vi "Acquire.vi"(8 "error in (no error)":errorcluster, 11 "Sensor in":refnum<class "Sensor.lvclass">) -> (0 "error out":errorcluster, 3 "Sensor out":refnum<class "Sensor.lvclass">)   [LabVIEW 2012, in "Sensor Definition.lvlib" / "Sensor.lvclass"]
uses:
  Sensor.lvclass
  Double Scalar SensorData.lvclass
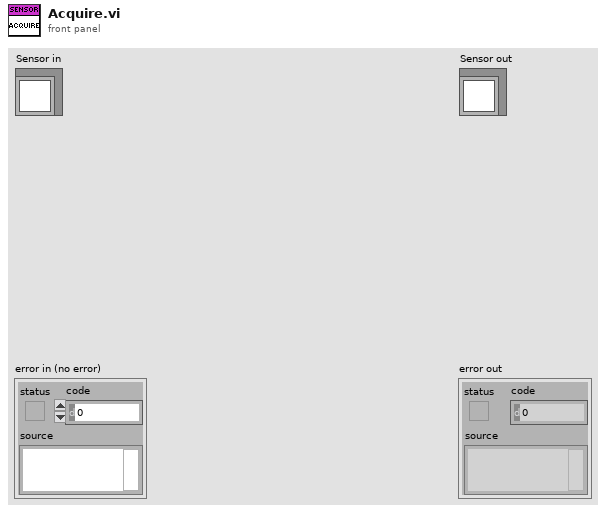
[diagram p1: front panel]
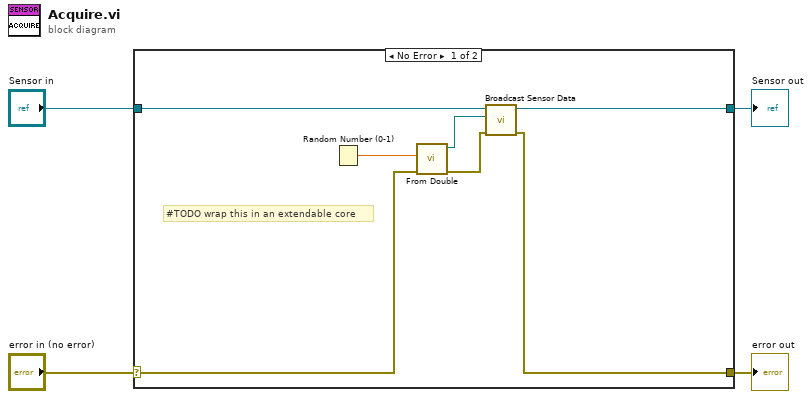
[diagram p0: block diagram]
diagram:
  n1 = case shown="No Error" "error in (no error)" {
    selector: "error in (no error)" -> [w6 w13]
    tunnel: [w9 w13] -> w3
    tunnel: [w10 w12] -> w1
    tunnel: "Sensor in" -> [w11 w12]
    frame No Error {
      # "#TODO wrap this in an extendable core"
      n2 = Random Number (0-1)() -> (number: 0 to 1=w7:dbl)
      n3 = call "From Double.vi"("error in (no error)"=w6, "Double"=w7) -> ("error out"=w5:errorcluster, "Double Scalar SensorData out"=w8:refnum<class "Double Scalar SensorData.lvclass">)  [unwired: 8 in]
      n4 = call "Broadcast Sensor Data.vi"("error in (no error)"=w5, "SensorData"=w8, "Sensor in"=w11) -> ("error out"=w9:errorcluster, "Sensor out"=w10:refnum<class "Sensor.lvclass">)  [unwired: 7 in]
    }
    frame Error {
    }
  }
  "error out" <- w3
  "Sensor out" <- w1
